vi "Windows_to_cygwin_path_conversion.vi"(11 "Windows path":path) -> (3 "Cygwin deata directory path":string)   [LabVIEW 2014]
panel:
  out "Path conv to string":string
  out "array of strings":string[](array[string])
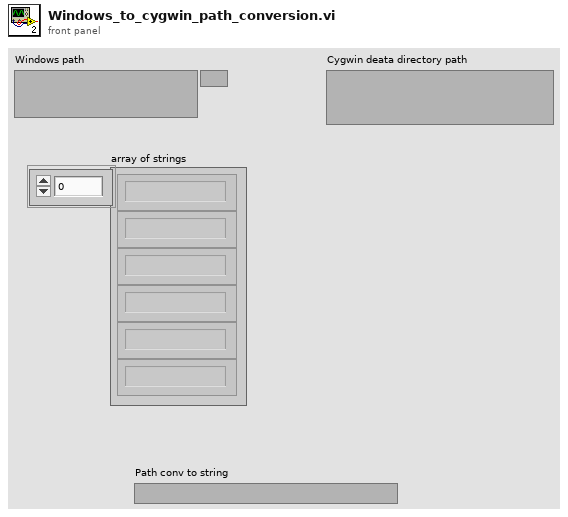
[diagram p1: front panel]
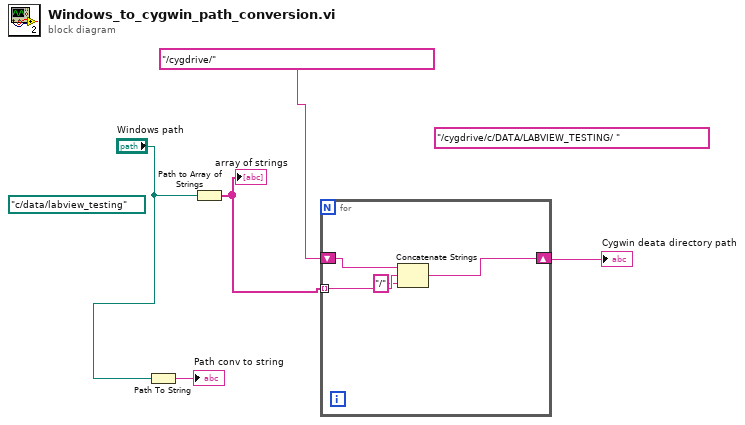
[diagram p0: block diagram]
diagram:
  (unwired) path "c:/data/labview_testing"
  (unwired) "/cygdrive/c/DATA/LABVIEW_TESTING/ " ("command line")
  n1 = Path To String(path="Windows path") -> (string=→"Path conv to string":string)
  n2 = Path to Array of Strings(0:"Windows path") -> (2:w5:string[])  [unwired: 1 out]
  "array of strings" <- w5
  n3 = for {
    tunnel: w5 -> [w8] mode=indexing
    shift-right: [w6] -> w3
    shift-left: "/cygdrive/" ("command line") -> [w9]
    n4 = Concatenate Strings(w9, w8, "/" ("string")) -> (w6:string)
  }
  "Cygwin deata directory path" <- w3
